vi "Read aux text file.vi"(8 "error in (no error)":errorcluster, 10 "Aux text file path":path, 11 "TomoConversion in":refnum<class "TomoConversion.lvclass">) -> (0 "error out":errorcluster, 3 "TomoConversion out":refnum<class "TomoConversion.lvclass">)   [LabVIEW 2012, in "TomoConversion.lvclass"]
uses:
  TomoConversion.lvclass
  TomoConversion.lvclass/TomoConversion.ctl
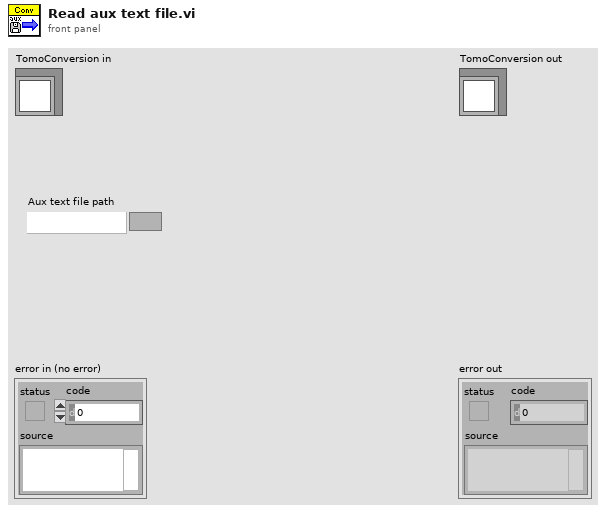
[diagram p1: front panel]
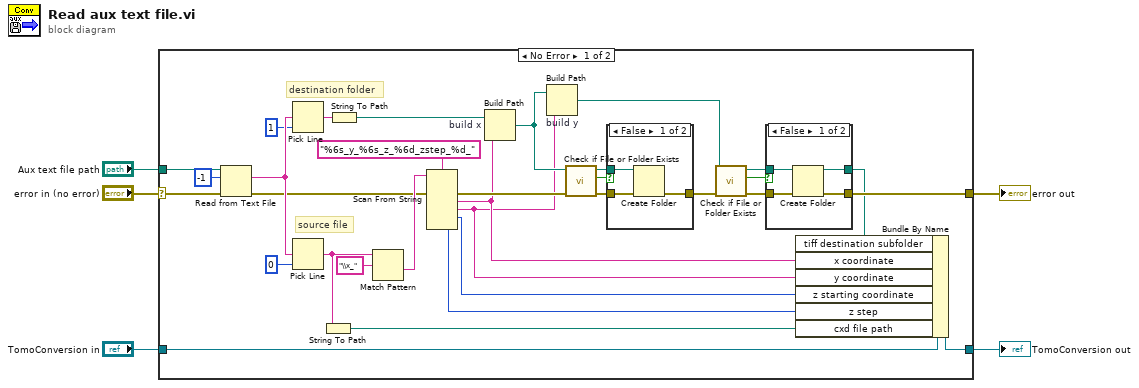
[diagram p0: block diagram]
diagram:
  n1 = case shown="No Error" "error in (no error)" {
    selector: "error in (no error)" -> [w35 w49]
    tunnel: [w16 w49] -> w4
    tunnel: [w14 w48] -> w2
    tunnel: "TomoConversion in" -> [w15 w48]
    tunnel: "Aux text file path" -> [w37 _]
    frame No Error {
      # "destination folder"
      # "source file"
      n2 = Read from Text File(file (use dialog)=w37, count=-1, error in=w35) -> (text=w34:string, error out=w26:errorcluster)  [unwired: 1 in, 2 out]
      n3 = Pick Line(multi-line string=w34, line index=1) -> (output string=w31:string)  [unwired: 1 in]
      n4 = Pick Line(multi-line string=w34, line index=0) -> (output string=w9:string)  [unwired: 1 in]
      n5 = String To Path(string=w9) -> (path=w8:path)
      n6 = String To Path(string=w31) -> (path=w30:path)
      n7 = Match Pattern(string=w9, regular expression="\\x_") -> (after substring=w28:string)  [unwired: 1 in, 3 out]
      n8 = Scan From String(format string="%6s_y_%6s_z_%6d_zstep_%d_", input string=w28, error in=w26) -> (error out=w25:errorcluster, output 1=w13:string, output 2=w12:string, output 3=w11:i32, output 4=w10:i32)  [unwired: 5 in, 2 out]
      n9 = Build Path "build x"(base path=w30, name or relative path=w13) -> (appended path=w21:path)
      n10 = Build Path "build y"(base path=w21, name or relative path=w12) -> (appended path=w7:path)
      n11 = call <vilib>:"Check if File or Folder Exists.vi"("error in (no error)"=w25, "path"=w21) -> ("error out"=w23:errorcluster, "file or folder exists?"=w24:bool, "dup path"=w22:path)  [unwired: 7 in]
      n12 = case shown="False" w24 {
        tunnel: w23 -> [w46 w47]
        tunnel: [w45 w47] -> w17
        tunnel: w22 -> [w44 _]
        frame False {
          n13 = Create Folder(path (use dialog)=w44, error in=w46) -> (error out=w45:errorcluster)  [unwired: 1 in, 2 out]
        }
        frame True {
        }
      }
      n14 = call <vilib>:"Check if File or Folder Exists.vi"("error in (no error)"=w17, "path"=w7) -> ("error out"=w19:errorcluster, "file or folder exists?"=w20:bool, "dup path"=w18:path)  [unwired: 7 in]
      n15 = case shown="False" w20 {
        tunnel: w19 -> [w41 w43]
        tunnel: [w40 w43] -> w16
        tunnel: w18 -> [w39 w42]
        tunnel: [w38 w42] -> w6
        frame False {
          n16 = Create Folder(path (use dialog)=w39, error in=w41) -> (created path=w38:path, error out=w40:errorcluster)  [unwired: 1 in, 1 out]
        }
        frame True {
        }
      }
      n17 = Bundle By Name(cluster=w15, "tiff destination subfolder"=w6, "x coordinate"=w13, "y coordinate"=w12, "z starting coordinate"=w11, "z step"=w10, "cxd file path"=w8) -> (w14:refnum<class "TomoConversion.lvclass">)
    }
    frame Error {
    }
  }
  "error out" <- w4
  "TomoConversion out" <- w2
